vi "Initialize.vi"(11 "MessengerMCPU in":refnum<class "MessengerMCPU.lvclass">) -> (3 "MessengerMCPU out":refnum<class "MessengerMCPU.lvclass">)   [LabVIEW 2019, in "MessengerM.lvlib" / "MessengerMCPU.lvclass"]
uses:
  MessengerMCPU.lvclass
  SubChannelCPU/SubChannelCPU.lvclass
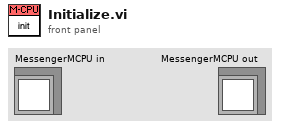
[diagram p1: front panel]
types:
  T1 = cluster{"GUID":string, "subchannel":refnum<class "SubChannelCPU.lvclass">}[]
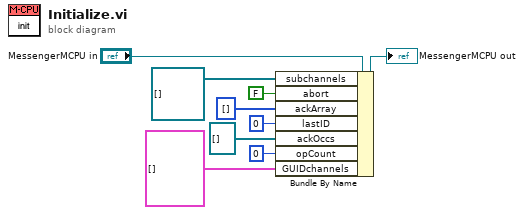
[diagram p0: block diagram]
diagram:
  n1 = Bundle By Name(cluster="MessengerMCPU in", "subchannels"=refnum<class "SubChannelCPU.lvclass">[] [], "abort"=FALSE, "ackArray"=u32[] [], "lastID"=u32 0, "ackOccs"=refnum<k4>[] [], "opCount"=u32 0, "GUIDchannels"=T1 []) -> (→"MessengerMCPU out":refnum<class "MessengerMCPU.lvclass">)
